vi "Write dest_vel.vi"(8 "error in (no error)":errorcluster, 10 "dest_vel":dbl, 11 "Robot in":refnum<class "Robot.lvclass">) -> (0 "error out":errorcluster, 3 "Robot out":refnum<class "Robot.lvclass">)   [LabVIEW 2018, in "Robot.lvclass"]
uses:
  Robot.lvclass
  Robot.lvclass/Robot.ctl
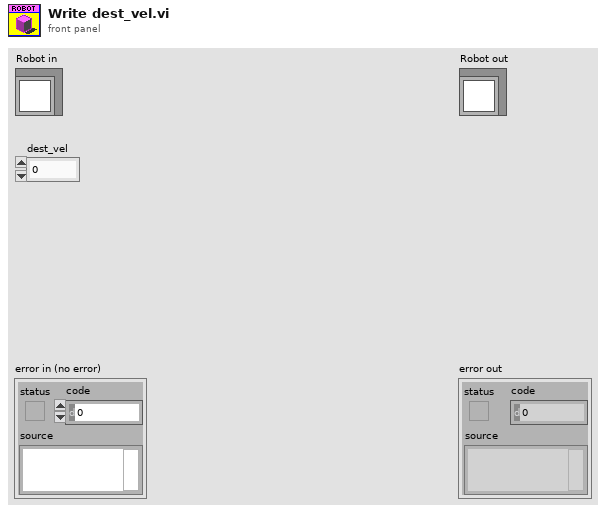
[diagram p1: front panel]
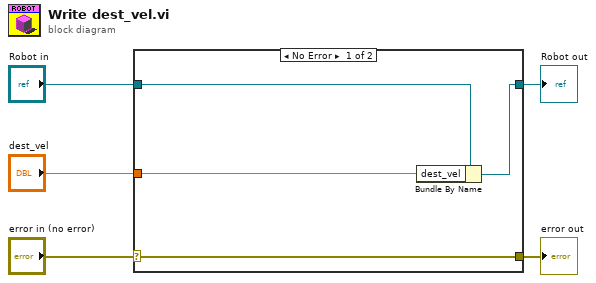
[diagram p0: block diagram]
diagram:
  n1 = case shown="No Error" "error in (no error)" {
    selector: "error in (no error)" -> [w9 w10]
    tunnel: [w9 w10] -> w4
    tunnel: [w7 w11] -> w2
    tunnel: "Robot in" -> [w8 w11]
    tunnel: "dest_vel" -> [w6 _]
    frame No Error {
      n2 = Bundle By Name(cluster=w8, "dest_vel"=w6) -> (w7:refnum<class "Robot.lvclass">)
    }
    frame Error {
    }
  }
  "error out" <- w4
  "Robot out" <- w2
